vi "ApplyInstrument.vi"(0 "Instrument":string, 1 "ITC ref":T1={"ITC"=0, "Signal"=enum."Sensor 3"}, 2 "Conversion Factor Fix\n1 V = ??":dbl=1.0, 3 "K2400 1":refnum<visa-resource-name>, 4 "Sweep Instrument":string(combo), 5 "Valin":dbl, 6 "Fix Instrument":string(combo), 9 "DAC number":u8, 11 "error in (no error)":errorcluster, 12 "K2400 2":refnum<visa-resource-name>, 13 "Conversion Factor Sweep\n1 V = ??":dbl=1.0, 14 "Lockin1":refnum<visa-resource-name>) -> (15 "error out":errorcluster)   [LabVIEW 2011]
uses:
  gumLV8p2/D/Labviewsoft/transport/GUMS/Kelvinox drivers/ITCAPPS - Copie.LLB/ITCSignal.ctl
  gumLV8p2/D/Labviewsoft/transport/GUMS/Kelvinox drivers/ITCAPPS - Copie.LLB/ITCSignals.ctl
  GlobalVar.vi
  monochromatorcontrol/perHandlemonochromator.vi
  users/nicolas/PHySpec-SDK-1.0.0/Labview-example/libPhyspec/libPhyspec.lvlib
panel:
  out "concatenated string":string
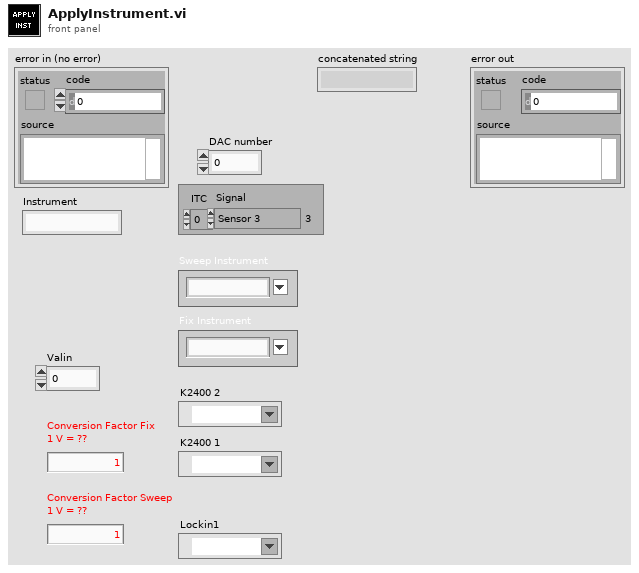
[diagram p1: front panel]
types:
  T1 = typedef "ITCSignal.ctl" = cluster{"ITC":u16, "Signal":T2}
  T2 = typedef "ITCSignals.ctl" = enum16{"Setpoint", "Sensor 1", "Sensor 2", "Sensor 3", "Needle Valve %", "Heater %"}
  T3 = cluster{"Power Stabilization":bool, "Laser Power [W]":dbl, "Power precision":dbl}
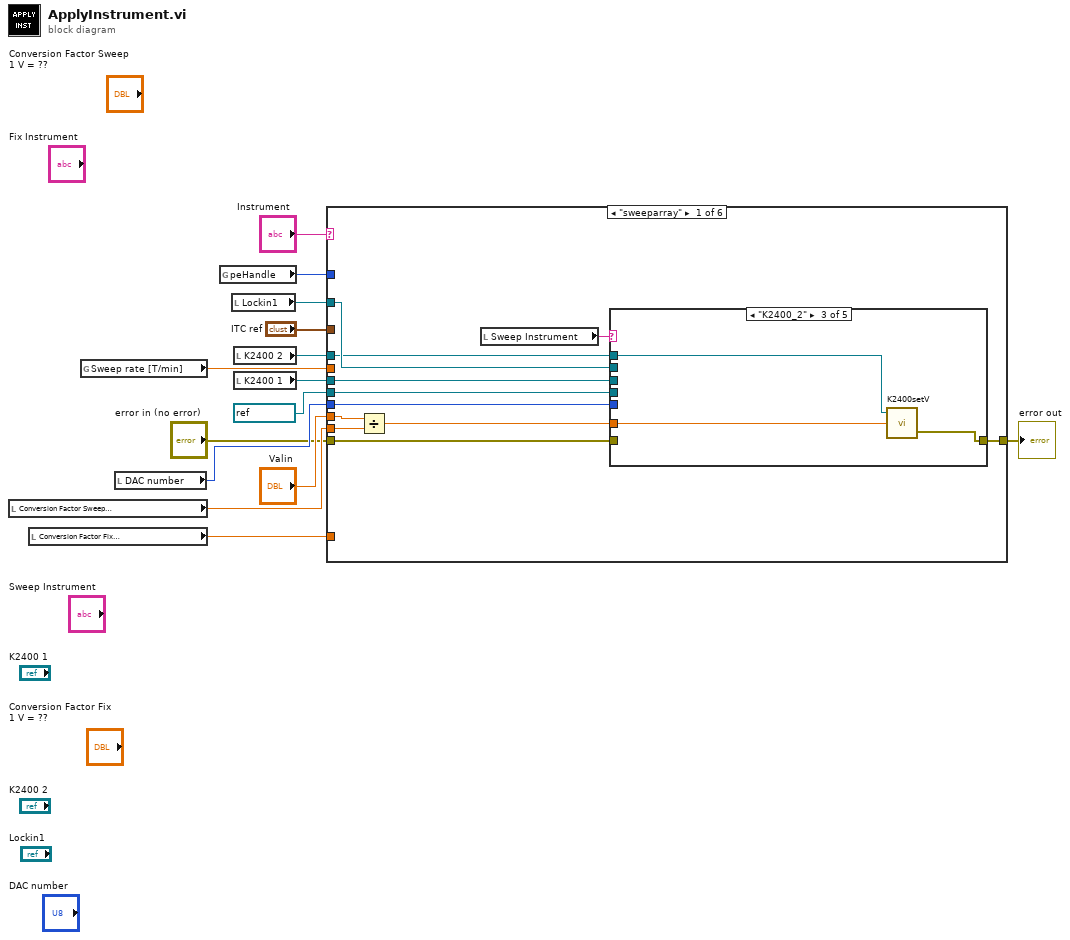
[diagram p0: block diagram]
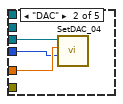
[diagram p3: hidden frame]
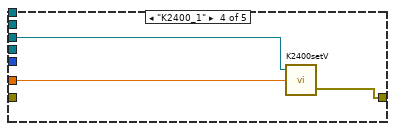
[diagram p4: hidden frame]
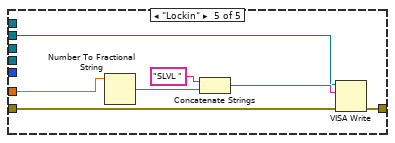
[diagram p5: hidden frame]
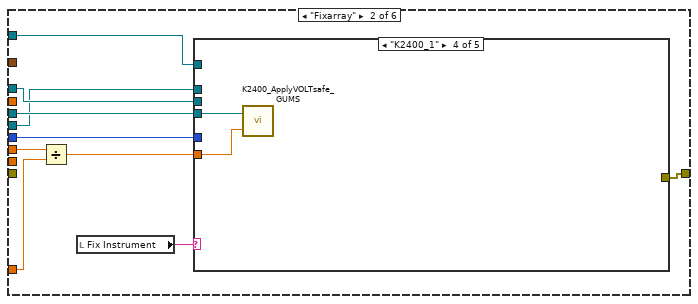
[diagram p6: hidden frame]
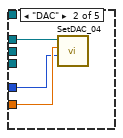
[diagram p8: hidden frame]
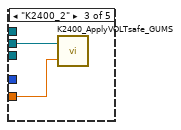
[diagram p9: hidden frame]
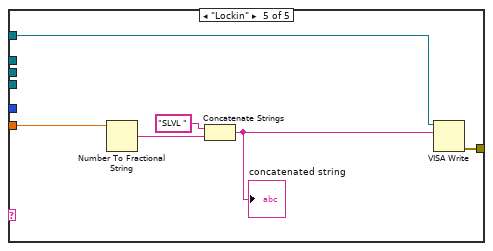
[diagram p10: hidden frame]
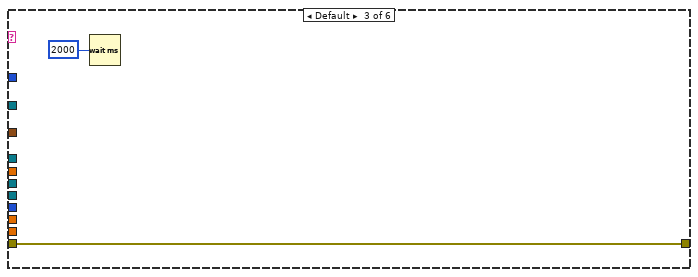
[diagram p11: hidden frame]
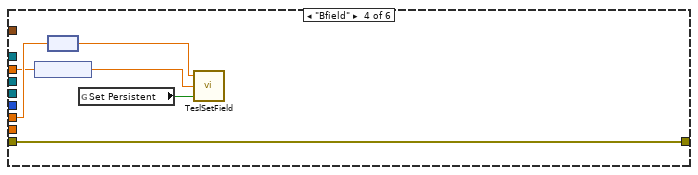
[diagram p12: hidden frame]
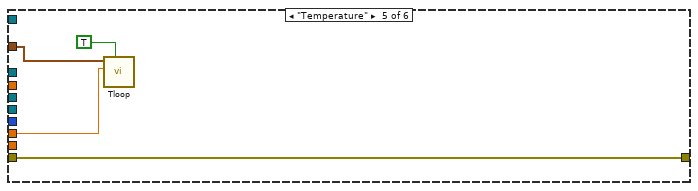
[diagram p13: hidden frame]
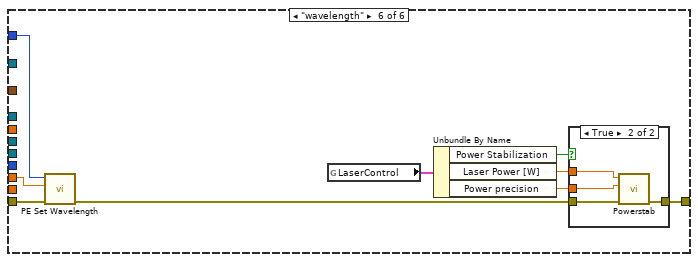
[diagram p14: hidden frame]
diagram:
  n1 = local read "Conversion Factor Sweep\n1 V = ??"() -> (w14:dbl)
  n2 = local read "Conversion Factor Fix\n1 V = ??"() -> (w13:dbl)
  n3 = global read "GlobalVar.vi" "Sweep rate [T/min]"() -> (w2:dbl)
  n4 = local read "DAC number"() -> (w12:u8)
  n5 = global read "perHandlemonochromator.vi" "peHandle"() -> (w1:u32)
  n6 = local read "Lockin1"() -> (w11:refnum<visa-resource-name>)
  n7 = local read "K2400 2"() -> (w10:refnum<visa-resource-name>)
  n8 = local read "K2400 1"() -> (w9:refnum<visa-resource-name>)
  n9 = case shown="\"sweeparray\"" "Instrument" {
    tunnel: "Valin" -> [w25 w51 _ w71 w76 w85]
    tunnel: "ITC ref" -> [_ _ _ _ w74 _]
    tunnel: w14 -> [w23 _ _ _ _ _]
    tunnel: w13 -> [_ w44 _ _ _ _]
    tunnel: w12 -> [w22 w49 _ _ _ _]
    tunnel: w11 -> [w21 w48 _ _ _ _]
    tunnel: w10 -> [w20 w47 _ _ _ _]
    tunnel: w9 -> [w19 w46 _ _ _ _]
    tunnel: w2 -> [_ _ _ w69 _ _]
    tunnel: "error in (no error)" -> [w17 _ w65 w68 w73 w83]
    tunnel: [w16 w43 w65 w68 w73 w79] -> w4
    tunnel: refnum<visa-resource-name> "COM1" ("RS232/ Optical Fiber") -> [w15 w42 _ _ _ _]
    tunnel: w1 -> [_ _ _ _ _ w84]
    frame "sweeparray" {
      n10 = Divide(x=w25, y=w23) -> (x/y=w24:dbl)
      n11 = local read "Sweep Instrument"() -> (w18:string)
      n12 = case shown="\"K2400_2\"" w18 {
        tunnel: w24 -> [_ w28 w31 w34 w38]
        tunnel: [_ _ w29 w33 w37] -> w16
        tunnel: w22 -> [_ w27 _ _ _]
        tunnel: w21 -> [_ _ _ _ w36]
        tunnel: w20 -> [_ _ w30 _ _]
        tunnel: w19 -> [_ _ _ w32 _]
        tunnel: w17 -> [_ _ _ _ w35]
        tunnel: w15 -> [_ w26 _ _ _]
        frame Default {
        }
        frame "DAC" {
          n13 = call "SetDAC_04.vi"("RS232/ Optical Fiber"=w26, "DATA (V)"=w28, "DAC nr"=w27) -> ()  [unwired: 2 in, 1 out]
        }
        frame "K2400_2" {
          n14 = call "K2400setV.vi"("Voltage target [V]"=w31, "VISA Resource Name"=w30) -> ("error out"=w29:errorcluster)  [unwired: 1 in, 1 out]
        }
        frame "K2400_1" {
          n15 = call "K2400setV.vi"("Voltage target [V]"=w34, "VISA Resource Name"=w32) -> ("error out"=w33:errorcluster)  [unwired: 1 in, 1 out]
        }
        frame "Lockin" {
          n16 = Number To Fractional String(number=w38) -> (F-format string=w41:string)  [unwired: 3 out]
          n17 = Concatenate Strings("SLVL " ("chaîne"), w41) -> (w39:string)
          n18 = VISA Write(VISA resource name=w36, write buffer=w39, error in (no error)=w35) -> (error out=w37:errorcluster)  [unwired: 2 out]
        }
      }
    }
    frame "Fixarray" {
      n19 = Divide(x=w51, y=w44) -> (x/y=w50:dbl)
      n20 = local read "Fix Instrument"() -> (w45:string)
      n21 = case shown="\"K2400_1\"" w45 {
        tunnel: w50 -> [_ w53 w55 w57 w61]
        tunnel: [_ _ _ _ w60] -> w43
        tunnel: w49 -> [_ w52 _ _ _]
        tunnel: w48 -> [_ _ _ _ w59]
        tunnel: w47 -> [_ _ w56 _ _]
        tunnel: w46 -> [_ _ _ w58 _]
        tunnel: w42 -> [_ w54 _ _ _]
        frame Default {
        }
        frame "DAC" {
          n22 = call "SetDAC_04.vi"("RS232/ Optical Fiber"=w54, "DATA (V)"=w53, "DAC nr"=w52) -> ()  [unwired: 2 in, 1 out]
        }
        frame "K2400_2" {
          n23 = call "K2400_ApplyVOLTsafe_GUMS.vi"("Voltage target [V]"=w55, "VISA Resource Name"=w56) -> ()  [unwired: 1 in]
        }
        frame "K2400_1" {
          n24 = call "K2400_ApplyVOLTsafe_GUMS.vi"("Voltage target [V]"=w57, "VISA Resource Name"=w58) -> ()  [unwired: 1 in]
        }
        frame "Lockin" {
          n25 = Number To Fractional String(number=w61) -> (F-format string=w64:string)  [unwired: 3 out]
          n26 = Concatenate Strings("SLVL " ("chaîne"), w64) -> (w62:string)
          "concatenated string" <- w62
          n27 = VISA Write(VISA resource name=w59, write buffer=w62) -> (error out=w60:errorcluster)  [unwired: 1 in, 2 out]
        }
      }
    }
    frame Default {
      n28 = Wait (ms)(milliseconds to wait=u32 2000) -> ()  [unwired: 1 out]
    }
    frame "Bfield" {
      n29 = node(w69) -> (w72:dbl[unit])
      n30 = node(w71) -> (w70:dbl[unit])
      n31 = global read "GlobalVar.vi" "Set Persistent"() -> (w67:bool)
      n32 = call "TeslSetField.vi"("Set Persistent"=w67, "Sweep rate"=w72, "Field required:"=w70) -> ()  [unwired: 1 in, 2 out]
    }
    frame "Temperature" {
      n33 = call "Tloop.vi"("ITCSignal"=w74, "T target [K]"=w76, "Regulate ?"=TRUE) -> ()  [unwired: 2 in, 2 out]
    }
    frame "wavelength" {
      n34 = call "PE Set Wavelength.vi"("error in (no error)"=w83, "wavelength"=w85, "peHandle"=w84) -> ("error out"=w80:errorcluster)  [unwired: 7 in, 1 out]
      n35 = global read "GlobalVar.vi" "LaserControl"() -> (w82:T3)
      n36 = Unbundle By Name(w82) -> ("Power Stabilization"=w81:bool, "Laser Power [W]"=w78:dbl, "Power precision"=w77:dbl)
      n37 = case shown="True" w81 {
        tunnel: w80 -> [w86 w90]
        tunnel: [w86 w89] -> w79
        tunnel: w78 -> [_ w88]
        tunnel: w77 -> [_ w87]
        frame False {
        }
        frame True {
          n38 = call "Powerstab.vi"("error out"=w90, "Power precision"=w87, "Laser Power [W]"=w88) -> ("error out 2"=w89:errorcluster)  [unwired: 7 in, 1 out]
        }
      }
    }
  }
  "error out" <- w4
